vi "Get SMO PGSQL Log Paths.vi"(8 "error in (no error)":errorcluster, 11 "Instrument.sample-registry":refnum<class "Instrument.sample-registry.lvclass">) -> (0 "error out":errorcluster, 2 "Paths":string, 3 "Instrument.sample-registry out":refnum<class "Instrument.sample-registry.lvclass">)   [LabVIEW 2019, in "Instrument.sample-registry.lvclass"]
uses:
  Instrument.sample-registry.lvclass
  <userlib>/LevyLab/Levylab Instruments/Instrument Types/VSource/Instrument.VSource.lvclass
  Typedefs/Instrument.sample-registry.getAll--Cluster.ctl
  <userlib>/LevyLab/LV-Data/LV-Data.PG/LV-Data.PGSQL.lvclass
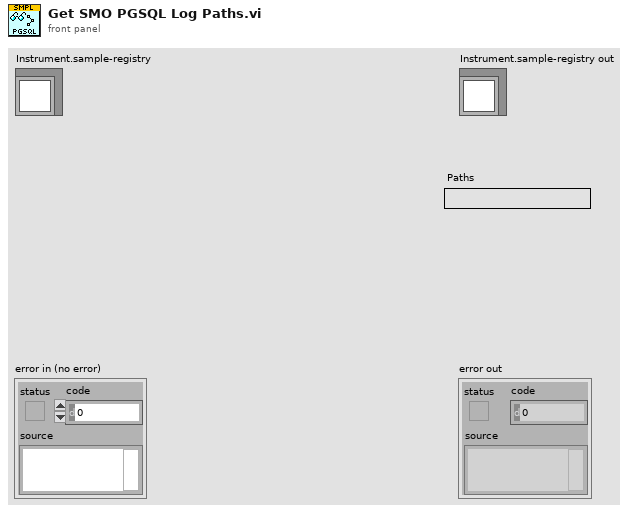
[diagram p1: front panel]
types:
  T1 = typedef "Instrument.sample-registry.lvclass/Instrument.sample-registry.getAll--Cluster.ctl" = cluster{"User":string, "Sample":string}
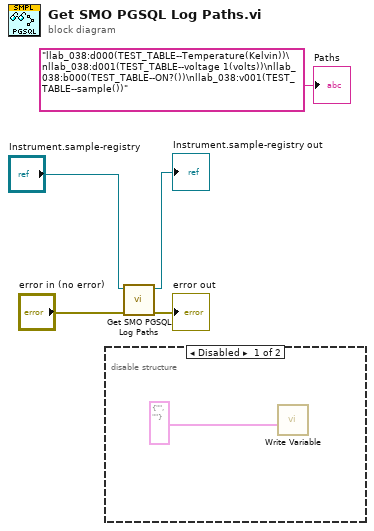
[diagram p0: block diagram]
diagram:
  n1 = disable-structure shown="Disabled" {
    frame Disabled {
      n2 = call <userlib>:"Write Variable.vi"("Data"=T1 {"User"="", "Sample"=""} ("getAll")) -> ()  [unwired: 8 in, 3 out]
    }
    frame Enabled {
    }
  }
  n3 = call-parent "Get SMO PGSQL Log Paths.vi"("error in (no error)"="error in (no error)", "Instrument in"="Instrument.sample-registry") -> ("error out"=→"error out":errorcluster, "Instrument out"=→"Instrument.sample-registry out":refnum<class "Instrument.sample-registry.lvclass">)  [unwired: 7 in, 1 out]
  "Paths" <- "llab_038:d000(TEST_TABLE--Temperature(Kelvin))\nllab_038:d001(TEST_TABLE--voltage 1(volts))\nllab_038:b000(TEST_TABLE--ON?())\nllab_038:v001(TEST_TABLE--sample())" ("Paths")
